vi "MyTestXL80.vi"() -> ()   [LabVIEW 2024]
uses:
  Library/Class/Renishaw-XL80/Renishaw-XL80.lvclass
panel:
  out "Iterations":i32
  in  "stop":bool
  out "GetLaserMeasurement":dbl format="%_8f"
  out "pStatus":i32(ring) items=["COUNT_OK"=0, "COUNT_ERROR"=1, "COUNT_TPIN_OCCURRED"=2, "COUNT_DATUMED"=4]
  out "Connect":bool
  out "Serial Number":string
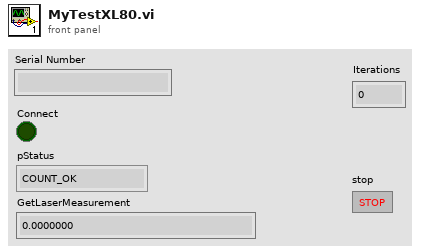
[diagram p1: front panel]
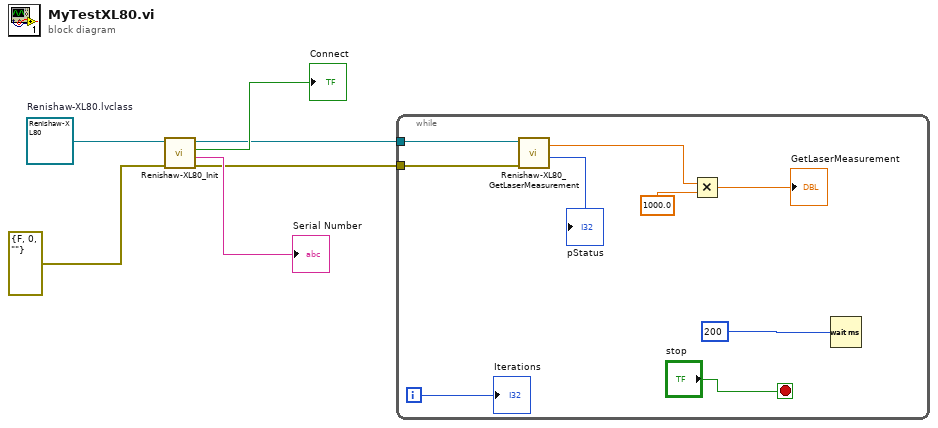
[diagram p0: block diagram]
diagram:
  w6 = refnum<class "Renishaw-XL80.lvclass"> refnum  # Renishaw-XL80.lvclass
  n1 = call-dynamic "Renishaw-XL80_Init.vi"("error in (no error)"=errorcluster {"status"=FALSE, "code"=0, "source"=""}, "Renishaw-XL80 in"=w6) -> ("error out"=w2:errorcluster, "Serial Number"=→"Serial Number":string, "Connect"=→"Connect":bool, "Renishaw-XL80 out"=w1:refnum<class "Renishaw-XL80.lvclass">)  [unwired: 6 in]
  n2 = while {
    tunnel: w2 -> [w14]
    tunnel: w1 -> [w13]
    i -> [w10]
    stop <- "stop" stop-if-true
    n3 = call-dynamic "Renishaw-XL80_GetLaserMeasurement.vi"("error in (no error)"=w14, "Renishaw-XL80 in"=w13) -> ("pStatus"=→"pStatus":i32, "GetLaserMeasurement"=w8:dbl)  [unwired: 6 in, 2 out]
    n4 = Multiply(x=w8, y=1000.0) -> (x*y=→"GetLaserMeasurement":dbl)
    n5 = Wait (ms)(milliseconds to wait=u32 200) -> ()  [unwired: 1 out]
    "Iterations" <- w10
  }
